vi "AI端口_电气.vi"() -> ()   [LabVIEW 2013]
panel:
  out "电气":tag="Dev1/ai3"
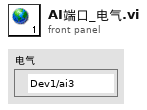
[diagram p1: front panel]
diagram:
